vi "PXI_Host_Bool_Write_NewMethod_Benchmark.vi"() -> ()   [LabVIEW 2018]
uses:
  <vilib>/Platform/TimedLoop/XDataNode/timing_clust.ctl
  <vilib>/Platform/TimedLoop/XDataNode/nitl_modes.ctl
  <vilib>/Platform/TimedLoop/XDataNode/wakeup.ctl
  cRIO RT/FPGA Bitfile Register Operations/Scalar IO Operations/Write Methods/Write Data Register/Instances/Write Boolean.vi
  cRIO RT/FPGA Bitfile Register Operations/Scalar IO Operations/Utilities/Find Register Offset.vi
  cRIO RT/FPGA Bitfile Register Operations/Scalar IO Operations/SubVIs/Check Register Data Store.vi
  cRIO RT/FPGA Bitfile Register Operations/Scalar IO Operations/Error Handling/Error 6001.vi
  cRIO RT/FPGA Bitfile Register Operations/Scalar IO Operations/Error Handling/Error 6000.vi
  cRIO RT/FPGA Bitfile Register Operations/Scalar IO Operations/Error Handling/Error 6002.vi
  cRIO RT/FPGA Bitfile Register Operations/Scalar IO Operations/Error Handling/Error 6006.vi
  <vilib>/FPGAPlugInAG/Dynamic/niLvFpga_Close_Dynamic.vi
  <vilib>/platform/TimedLoop/XDataNode/XDataNode.xnode
  <vilib>/rvi/interface/nirviCloseFPGA/nirviCloseFPGA.xnode
  cRIO RT/FPGA Bitfile Register Operations/Scalar IO Operations/FPGA Register IO.lvlib
  <vilib>/Platform/TimedLoop/XDataNode/XDNodeRunTimeDep.lvlib
panel:
  out "Waveform Graph":dbl[](graph)
  out "Maximum(s)":dbl
  out "Standard deviation":dbl
  out "error out":errorcluster
  out "Execution time (s)":dbl
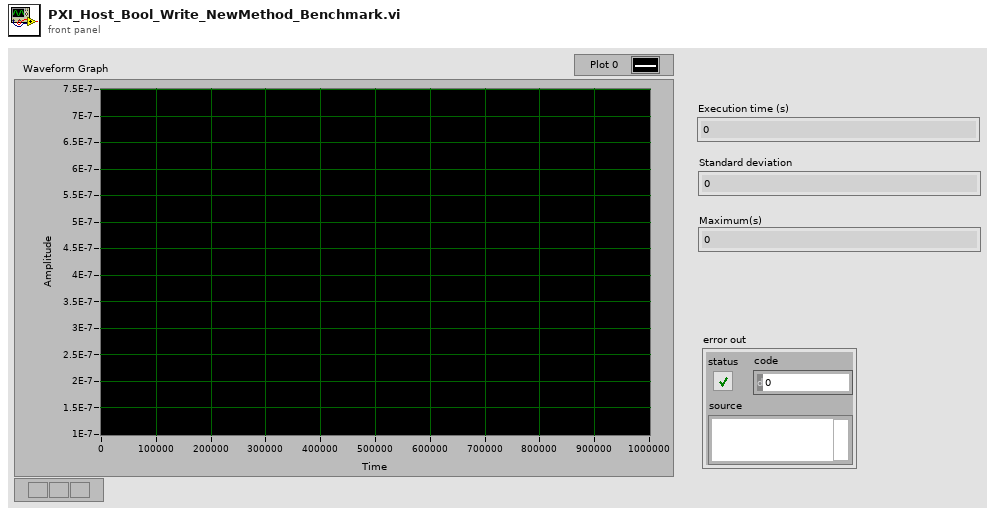
[diagram p1: front panel]
types:
  T1 = typedef "XDNodeRunTimeDep.lvlib/timing_clust.ctl" = cluster{"Expected End [f-1]":u64, "Actual End [f-1]":u64, "Finished Late? [f-1]":bool, "Expected End [i-1]":u64, "Actual End [i-1]":u64, "Finished Late? [i-1]":bool, "Expected Start [i]":u64, "Actual Start [i]":u64, "Expected Start [f]":u64, "Actual Start [f]":u64, "Source Name":string, "Structure Name":string, "Period":i64, "Deadline":i64, "Offset":i64, "Start":i64, "Priority":i32, "Timeout":i32, "Mode":T2, "Wakeup Reason":T3, "Error":errorcluster, "Source Type":string, "Secondary Source Type":string, "Global End Time":u64, "Global Start Time":u64, "Frame Duration":u64, "Iteration Duration":u64, "Assigned CPU":i32, "I/O Scan Engine Mode":u32}
  T2 = typedef "XDNodeRunTimeDep.lvlib/nitl_modes.ctl" = enum32{"No Change", "Process missed periods, maintain original phase", "Discard missed periods, maintain original phase", "Process missed periods, ignore original phase", "Discard missed periods, ignore original phase"}
  T3 = typedef "XDNodeRunTimeDep.lvlib/wakeup.ctl" = enum32{"Normal", "Aborted", "Asynchronous wakeup", "Timing source error", "Timed loop error", "Timeout"}
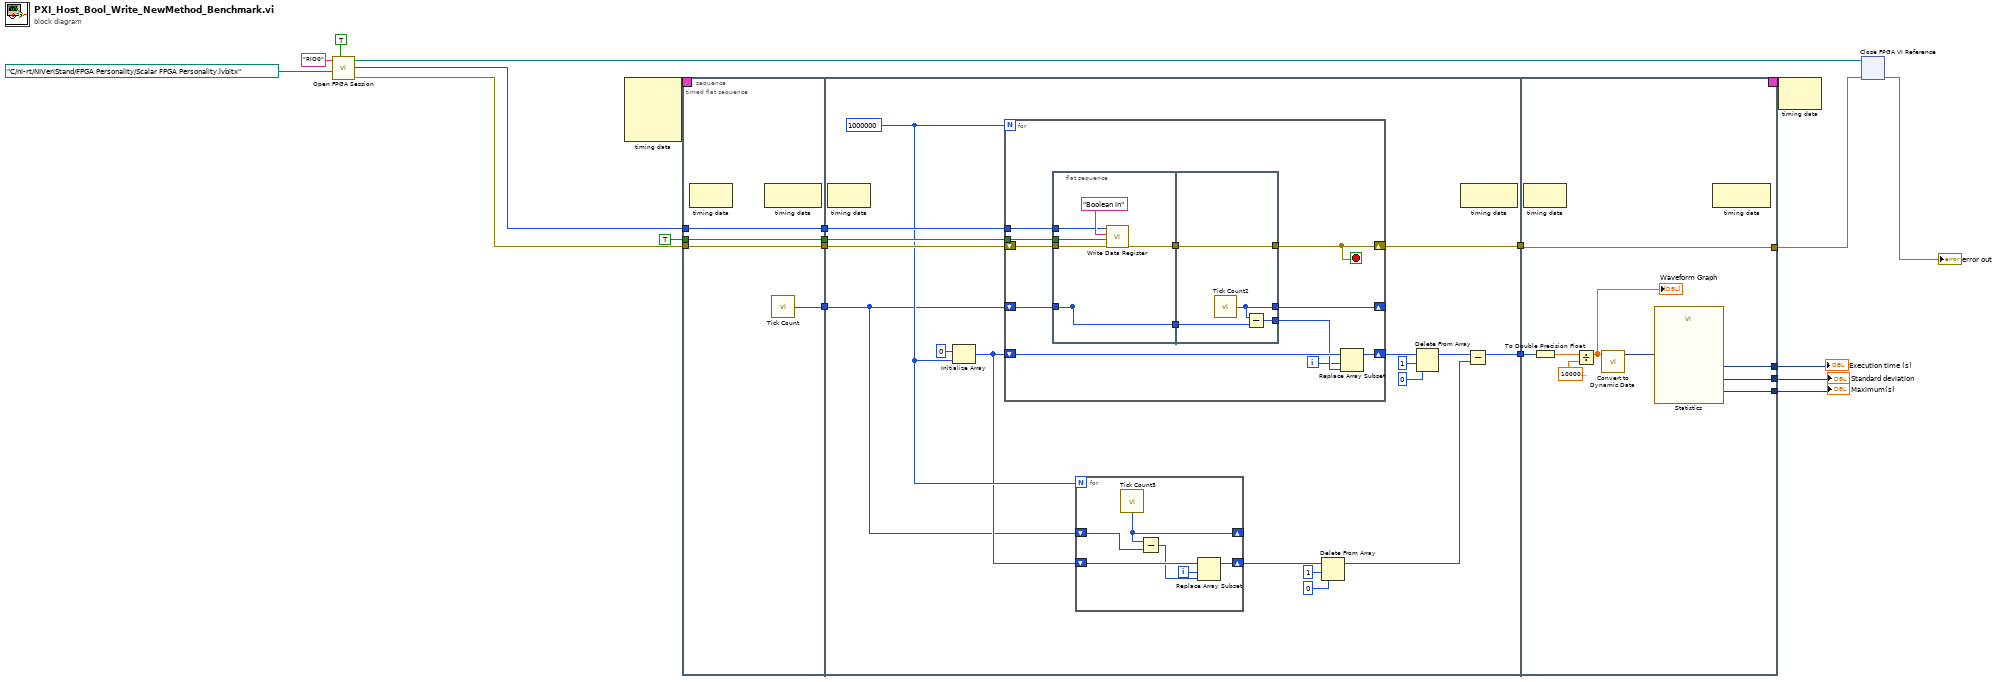
[diagram p0: block diagram]
diagram:
  n1 = call "Open FPGA Session.vi"("run when loaded (T)"=TRUE, "bitfile path"=path "C:/ni-rt/NIVeriStand/FPGA Personality/Scalar FPGA Personality.lvbitx", "device address"="RIO0") -> ("error out"=w10:errorcluster, "session out"=w14:u32, "bitfile reference out"=w9:refnum<k20>)  [unwired: 6 in]
  n2 = node-c288() -> (w5:T1)  [unwired: 4 in]
  n3 = timed-sequence {
    timing: w5 -> [_]
    timing-out: [_] -> w4
    tunnel: w14 -> [w27]
    tunnel: w10 -> [w26]
    tunnel: TRUE -> [w25]
    tunnel: [w20] -> w8
    tunnel: [w17] -> w3
    tunnel: [w16] -> w2
    tunnel: [w15] -> w1
    n4 = timed-flat-sequence {
      tunnel: w27 -> [w31]
      tunnel: [w31] -> w24
      tunnel: w26 -> [w30]
      tunnel: [w30] -> w23
      tunnel: w25 -> [w29]
      tunnel: [w29] -> w22
      tunnel: [w28] -> w19
      tunnel: w24 -> [w50]
      tunnel: w23 -> [w49]
      tunnel: [w48] -> w21
      tunnel: w22 -> [w47]
      tunnel: w19 -> [w37]
      tunnel: [w35] -> w18
      tunnel: w21 -> [w89]
      tunnel: [w89] -> w20
      tunnel: w18 -> [w88]
      tunnel: [w86] -> w17
      tunnel: [w83] -> w16
      tunnel: [w82] -> w15
      frame #0 {
        n5 = node-c288() -> ()  [unwired: 1 in, 1 out]
        n6 = node-c288() -> ()  [unwired: 1 in, 1 out]
        n7 = call "Tick Count"() -> ("Tick Count(Ticks)"=w28:u32)
      }
      frame #1 {
        w39 = 1000000
        n8 = node-c288() -> ()  [unwired: 1 in, 1 out]
        n9 = Initialize Array(u32 0, w39) -> (w38:u32[])
        n10 = for {
          N: w39 -> [_]
          tunnel: w50 -> [w69]
          tunnel: w47 -> [w68]
          shift-right: [w66] -> _
          shift-left: w37 -> [w65]
          shift-right: [w61] -> w45
          shift-left: w38 -> [w63]
          shift-right: [w59] -> w48
          shift-left: w49 -> [w70]
          i -> [w60]
          stop <- w59 stop-if-true
          n11 = flat-sequence {
            tunnel: w70 -> [w75]
            tunnel: w69 -> [w73]
            tunnel: w68 -> [w72]
            tunnel: [w76] -> w67
            tunnel: [w71] -> _
            tunnel: w65 -> [w71]
            tunnel: [w71] -> w64
            tunnel: [w80] -> w59
            tunnel: w67 -> [w80]
            tunnel: [w79] -> w66
            tunnel: w64 -> [w78]
            tunnel: [w77] -> w62
            frame #0 {
              n12 = call-poly "Write Data Register.vi"("error in"=w75, "value in"=w72, "register name"="Boolean in", "session in"=w73) -> ("error out"=w76:errorcluster)  [unwired: 6 in, 1 out]
            }
            frame #1 {
              n13 = call "Tick Count2"() -> ("Tick Count(Ticks)"=w79:u32)
              n14 = Subtract(x=w79, y=w78) -> (x-y=w77:u32)
            }
          }
          n15 = Replace Array Subset(array=w63, new element=w62, index=w60) -> (w61:u32[])
        }
        n16 = for {
          N: w39 -> [_]
          shift-right: [w51] -> w40
          shift-left: w38 -> [w54]
          shift-right: [w56] -> _
          shift-left: w37 -> [w55]
          i -> [w52]
          n17 = call "Tick Count3"() -> ("Tick Count(Ticks)"=w56:u32)
          n18 = Subtract(x=w56, y=w55) -> (x-y=w53:u32)
          n19 = Replace Array Subset(array=w54, new element=w53, index=w52) -> (w51:u32[])
        }
        n20 = Delete From Array(array=w40, length=1, index=0) -> (array with subset deleted=w34:u32[])  [unwired: 1 out]
        n21 = Delete From Array(array=w45, length=1, index=0) -> (array with subset deleted=w36:u32[])  [unwired: 1 out]
        n22 = node-c288() -> ()  [unwired: 1 in, 1 out]
        n23 = Subtract(x=w36, y=w34) -> (x-y=w35:u32[])
      }
      frame #2 {
        n24 = node-c288() -> ()  [unwired: 1 in, 1 out]
        n25 = To Double Precision Float(number=w88) -> (double precision float=w85:dbl[])
        n26 = Divide(x=w85, y=1000000000.0) -> (x/y=w81:dbl[])
        "Waveform Graph" <- w81
        n27 = call "Convert to Dynamic Data"("Array"=w81) -> ("Dynamic Data Type"=w87:dynamicdata)  [unwired: 3 in]
        n28 = call "Statistics"("Signals"=w87) -> ("Standard Dev"=w83:dynamicdata, "Arithmetic Mean"=w86:dynamicdata, "Maximum"=w82:dynamicdata)  [unwired: 23 in, 1 out]
        n29 = node-c288() -> ()  [unwired: 1 in, 1 out]
      }
    }
  }
  "Execution time (s)" <- w3
  "Standard deviation" <- w2
  "Maximum(s)" <- w1
  n30 = node-c288(w4) -> ()  [unwired: 1 out]
  n31 = xnode "Close FPGA VI Reference"("FPGA VI Reference In"=w9, "error in"=w8) -> ("error out"=→"error out":errorcluster)
